vi "TCP Read.vi"(8 "error in":errorcluster, 9 "timeout":i32, 10 "bytes to read":i32, 11 "connection ID":refnum<k5>) -> (0 "error out":errorcluster, 1 "timed out?":bool, 2 "data":u8[](array[numeric]), 3 "connection ID out":refnum<k5>)   [LabVIEW 2021, in "TCP Shared Components.lvlib"]
doc: "This function reads a TCP packet from the bus and checks for errors. It is a wrapper for standard functionality."
uses:
  TCP Shared Components.lvlib
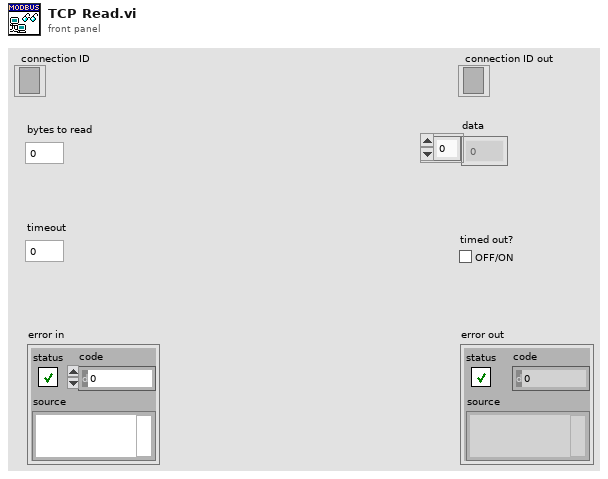
[diagram p1: front panel]
types:
  T1 = enum16{"Standard", "Buffered", "CRLF", "Immediate"}
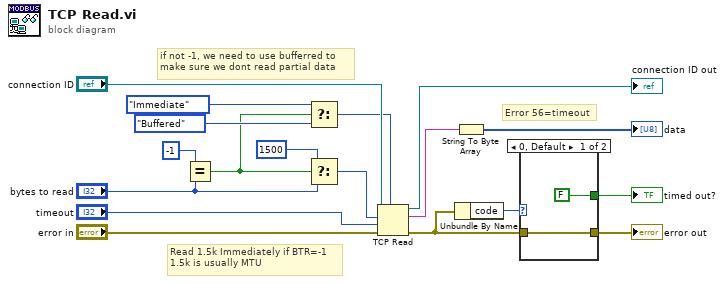
[diagram p0: block diagram]
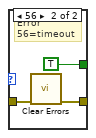
[diagram p2: hidden frame]
diagram:
  # "Error 56=timeout"
  # "Read 1.5k Immediately if BTR=-1\n1.5k is usually MTU"
  # "if not -1, we need to use bufferred to\nmake sure we dont read partial data"
  n1 = Equal?(x=-1, y="bytes to read") -> (x = y?=w7:bool)
  n2 = Select(t=T1."Immediate" ("mode (standard)"), s=w7, f=T1."Buffered" ("mode (standard)")) -> (s? t:f=w8:T1)
  n3 = Select(t=1500, s=w7, f="bytes to read") -> (s? t:f=w6:i32)
  n4 = TCP Read(connection ID="connection ID", bytes to read=w6, error in (no error)="error in", 7:w8, 9:"timeout") -> (connection ID out=→"connection ID out":refnum<k5>, data out=w3:string, error out=w4:errorcluster)
  n5 = Unbundle By Name(w4) -> ("code"=w2:i32)
  n6 = String To Byte Array(string=w3) -> (unsigned byte array=→"data":u8[])
  n7 = case shown="0, Default" w2 {
    tunnel: w4 -> [w20 w22]
    tunnel: [w20 w21] -> w13
    tunnel: [FALSE TRUE] -> w12
    frame 0, Default {
    }
    frame 56 {
      # "Error 56=timeout"
      n8 = call <vilib>:"Clear Errors.vi"("error in (no error)"=w22) -> ("error out"=w21:errorcluster)  [unwired: 5 in, 1 out]
    }
  }
  "error out" <- w13
  "timed out?" <- w12
